vi "AddTreeItem.vi"(0 "filenames":string[](array[string]), 1 "folders":string[](array[string]), 2 "ParentTag":string, 3 "CtlRef 2":refnum<vi>) -> ()   [LabVIEW 2010]
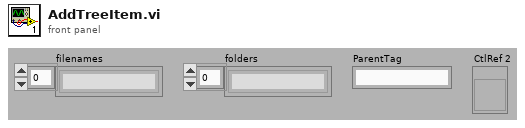
[diagram p1: front panel]
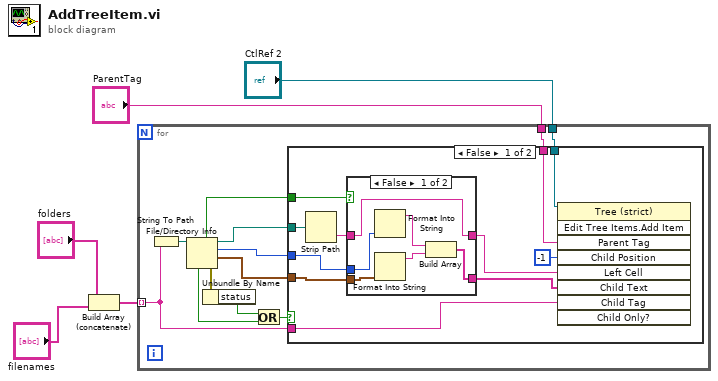
[diagram p0: block diagram]
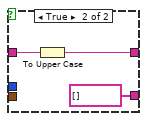
[diagram p2: hidden frame]
diagram:
  n1 = Build Array (concatenate)("folders", "filenames") -> (w1:string[])
  n2 = for {
    tunnel: "CtlRef 2" -> [w17]
    tunnel: w1 -> [w15] mode=indexing
    tunnel: "ParentTag" -> [w16]
    n3 = String To Path(string=w15) -> (path=w14:path)
    n4 = File/Directory Info(path=w14) -> (path out=w12:path, directory=w13:bool, size=w11:i64, last mod=w10:timestamp, error out=w9:errorcluster, shortcut=w7:bool)  [unwired: 1 in, 1 out]
    n5 = Unbundle By Name(w9) -> ("status"=w8:bool)
    n6 = Or(x=w8, y=w7) -> (x .or. y?=w6:bool)
    n7 = case shown="False" w6 {
      tunnel: w17 -> [w28 _]
      tunnel: w16 -> [w26 _]
      tunnel: w15 -> [w25 _]
      tunnel: w13 -> [w24 _]
      tunnel: w12 -> [w23 _]
      tunnel: w11 -> [w20 _]
      tunnel: w10 -> [w19 _]
      frame False {
        n8 = Strip Path(path=w23) -> (name=w22:string)  [unwired: 1 out]
        n9 = case shown="False" w24 {
          tunnel: w22 -> [w29 w37]
          tunnel: [w29 w36] -> w21
          tunnel: w20 -> [w34 _]
          tunnel: w19 -> [w33 _]
          tunnel: [w30 string[] []] -> w18
          frame False {
            n10 = Format Into String(w34) -> (resulting string=w32:string)  [unwired: 3 in, 1 out]
            n11 = Format Into String(w33) -> (resulting string=w31:string)  [unwired: 3 in, 1 out]
            n12 = Build Array(w32, w31) -> (w30:string[])
          }
          frame True {
            n13 = To Upper Case(1:w37) -> (0:w36:string)
          }
        }
        n14 = invoke class="Tree (strict)" method="Edit Tree Items.Add Item"(reference=w28, "Parent Tag"=w26, "Child Position"=-1, "Left Cell"=w21, "Child Text"=w18, "Child Tag"=w25) -> ()  [unwired: 3 in, 9 out]
      }
      frame True {
      }
    }
  }
